vi "updateDisplay.vi"(8 "error in (no error)":errorcluster, 11 "ScriptEditorV2 in":refnum<class "ScriptEditorV2.lvclass">) -> (0 "error out":errorcluster, 3 "ScriptEditorV2 out":refnum<class "ScriptEditorV2.lvclass">)   [LabVIEW 2009, in "Views.lvlib" / "ScriptEditor.lvlib" / "ScriptEditorV2.lvclass"]
uses:
  ScriptEditorV2.lvclass
  ScriptEditorV2.lvclass/ScriptEditorV2.ctl
  Tools/Scripting/ScriptingEvent/ScriptEventList/ScriptEventList.lvclass
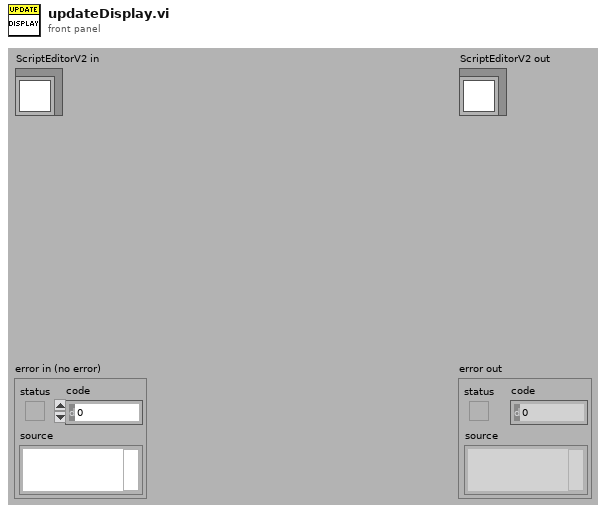
[diagram p1: front panel]
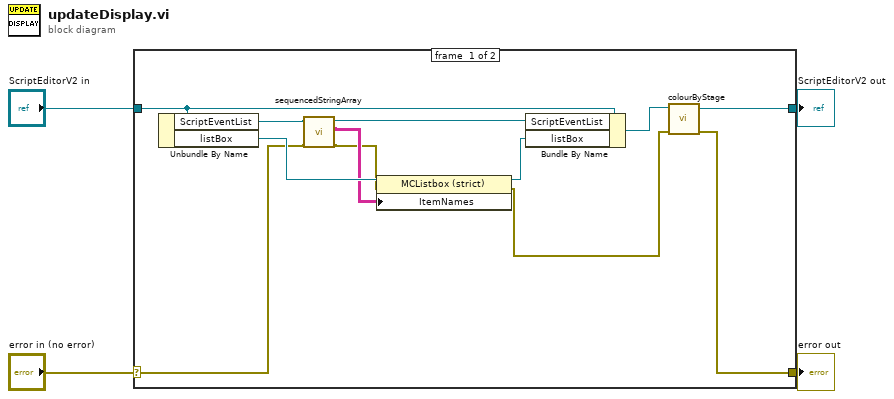
[diagram p0: block diagram]
diagram:
  n1 = case shown="No Error" "error in (no error)" {
    selector: "error in (no error)" -> [w13 w18]
    tunnel: [w5 w18] -> w3
    tunnel: [w8 w17] -> w1
    tunnel: "ScriptEditorV2 in" -> [w16 w17]
    frame #0 {
      n2 = Unbundle By Name(w16) -> ("ScriptEventList"=w12:refnum<class "ScriptEventList.lvclass">, "listBox"=w15:refnum<vi>)
      n3 = call "sequencedStringArray.vi"("error in (no error)"=w13, "ScriptEventList in"=w12) -> ("error out"=w9:errorcluster, "eventStringArray"=w10:string[][], "ScriptEventList out"=w11:refnum<class "ScriptEventList.lvclass">)  [unwired: 7 in]
      n4 = property class="MCListbox (strict)"(reference=w15, error in=w9, "ItemNames"=w10) -> (reference out=w14:refnum<vi>, error out=w6:errorcluster)
      n5 = Bundle By Name(cluster=w16, "ScriptEventList"=w11, "listBox"=w14) -> (w7:refnum<class "ScriptEditorV2.lvclass">)
      n6 = call "colourByStage.vi"("error in (no error)"=w6, "ScriptEditorV2 in"=w7) -> ("error out"=w5:errorcluster, "ScriptEditorV2 out"=w8:refnum<class "ScriptEditorV2.lvclass">)  [unwired: 8 in]
    }
    frame #1 {
    }
  }
  "error out" <- w3
  "ScriptEditorV2 out" <- w1
